vi "Reference Table Extractor.vi"(11 "distance":dbl(slide) scale=0.0..6.0 scale format="%3d") -> (0 "Shooting Range":bool, 1 "Error Margin":dbl, 2 "Catapult Move\nAngle":i32, 3 "RPM":i32)   [LabVIEW 2013]
uses:
  Reference Global.vi
panel:
  out "Distance on\nLookup Table":string
  out "Element Number":i32
  # "This is in Metrics"
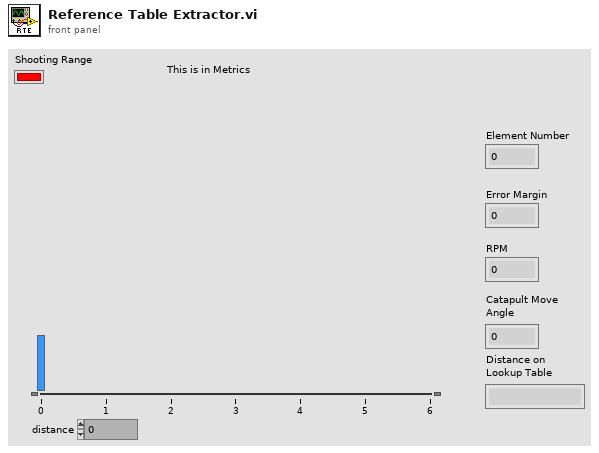
[diagram p1: front panel]
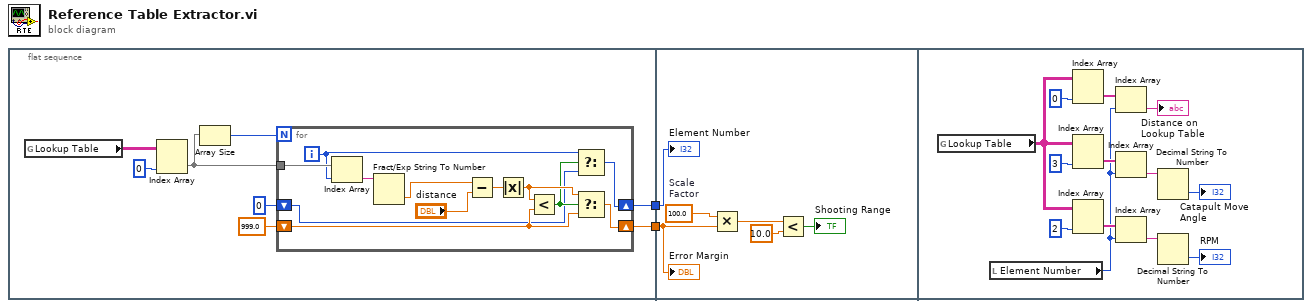
[diagram p0: block diagram]
diagram:
  n1 = flat-sequence {
    tunnel: [w8] -> w2
    tunnel: [w7] -> w1
    tunnel: w2 -> [w23]
    tunnel: w1 -> [w24]
    frame #0 {
      n2 = global read "Reference Global.vi" "Lookup Table"() -> (w3:string[][])
      n3 = Index Array(array=w3, index (col)=0 ("disabled index (col)")) -> (element=w4:string[])  [unwired: 1 in]
      n4 = Array Size(array=w4) -> (size(s)=w9:i32)
      n5 = for {
        N: w9 -> [_]
        tunnel: w4 -> [w22]
        shift-right: [w17] -> w8
        shift-left: 999.0 -> [w18]
        shift-right: [w15] -> w7
        shift-left: 0 -> [w14]
        i -> [w13]
        n6 = Index Array(array=w22, index=w13) -> (element=w12:string)
        n7 = Fract/Exp String To Number(string=w12) -> (number=w11:dbl)  [unwired: 3 in, 1 out]
        n8 = Subtract(x=w11, y="distance") -> (x-y=w21:dbl)
        n9 = Absolute Value(x=w21) -> (abs(x)=w19:dbl)
        n10 = Less?(x=w19, y=w18) -> (x < y?=w16:bool)
        n11 = Select(t=w13, s=w16, f=w14) -> (s? t:f=w15:i32)
        n12 = Select(t=w19, s=w16, f=w18) -> (s? t:f=w17:dbl)
      }
    }
    frame #1 {
      w28 = 100.0  # Scale Factor
      n13 = Multiply(x=w28, y=w23) -> (x*y=w27:dbl)
      n14 = Less?(x=w27, y=10.0) -> (x < y?=→"Shooting Range":bool)
      "Error Margin" <- w23
      "Element Number" <- w24
    }
    frame #2 {
      n15 = global read "Reference Global.vi" "Lookup Table"() -> (w33:string[][])
      n16 = local read "Element Number"() -> (w31:i32)
      n17 = Index Array(array=w33, index (col)=0 ("disabled index (col)")) -> (element=w30:string[])  [unwired: 1 in]
      n18 = Index Array(array=w33, index (col)=3 ("disabled index (col)")) -> (element=w38:string[])  [unwired: 1 in]
      n19 = Index Array(array=w33, index (col)=2 ("disabled index (col)")) -> (element=w39:string[])  [unwired: 1 in]
      n20 = Index Array(array=w30, index=w31) -> (element=→"Distance on\nLookup Table":string)
      n21 = Index Array(array=w38, index=w31) -> (element=w35:string)
      n22 = Index Array(array=w39, index=w31) -> (element=w37:string)
      n23 = Decimal String To Number(string=w35) -> (number=→"Catapult Move\nAngle":i32)  [unwired: 2 in, 1 out]
      n24 = Decimal String To Number(string=w37) -> (number=→"RPM":i32)  [unwired: 2 in, 1 out]
    }
  }
